vi "Seconds_To_String.vi"(1 "Seconds":dbl) -> (0 "Output String":string)   [LabVIEW 2011]
doc: "This VI returns a time string corresponding to the \"Seconds\" parameter in the form of H:MM:SS."
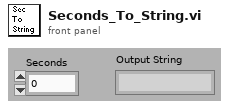
[diagram p1: front panel]
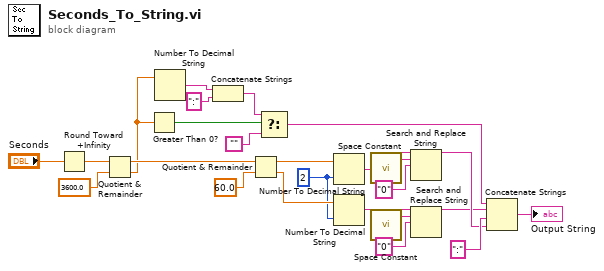
[diagram p0: block diagram]
diagram:
  w1 = i16 2 ("width (-)")
  n1 = Round Toward +Infinity(x="Seconds") -> (ceil(x): smallest int >= x=w14:dbl)
  n2 = Quotient & Remainder(x=w14, y=3600.0) -> (x-y*floor(x/y)=w13:dbl, floor(x/y)=w12:dbl)
  n3 = Greater Than 0?(x=w12) -> (x > 0?=w2:bool)
  n4 = Number To Decimal String(number=w12) -> (decimal integer string=w9:string)  [unwired: 1 out]
  n5 = Concatenate Strings(w9, ":" ("string")) -> (w7:string)
  n6 = Quotient & Remainder(x=w13, y=60.0) -> (x-y*floor(x/y)=w25:dbl, floor(x/y)=w24:dbl)
  n7 = Select(t=w7, s=w2, f="") -> (s? t:f=w10:string)
  n8 = Number To Decimal String(number=w25, width (-)=w1) -> (decimal integer string=w20:string)
  n9 = Number To Decimal String(number=w24, width (-)=w1) -> (decimal integer string=w4:string)
  n10 = call <vilib>:"Space Constant.vi"() -> ("String"=w22:string)
  n11 = call <vilib>:"Space Constant.vi"() -> ("String"=w6:string)
  n12 = Search and Replace String(input string=w20, search string=w22, replace string="0" ("replace string (\"\")")) -> (result string=w19:string)  [unwired: 1 in, 7 out]
  n13 = Search and Replace String(input string=w4, search string=w6, replace string="0" ("replace string (\"\")")) -> (result string=w3:string)  [unwired: 1 in, 7 out]
  n14 = Concatenate Strings(w10, w3, ":" ("string"), w19) -> (→"Output String":string)
